vi "test_erp42.vi"(11 "Data":T3={"Drive_value"={"F/B"=enum."N", "Speed"=0, "Steer"=-82, "A/M"=enum."Auto", "Brake"=0}} {"Drive_value"."Brake" scale=0.0..200.0; "Drive_value"."Steer" scale=-2000.0..2000.0; "Drive_value"."Speed" scale=0.0..100.0}) -> (2 "ERP_Receive":T2, 3 "data val":bool)   [LabVIEW 2019]
uses:
  Ctrl/data.ctl
  Ctrl/erp42_receive_packet.ctl
panel:
  in  "AGV cfg":T1={"Port"="COM32", "speed limits"={"limit_linear-v"=0.5, "limit_angular-v"=0.7999999999999999}}
  in  "정지":bool
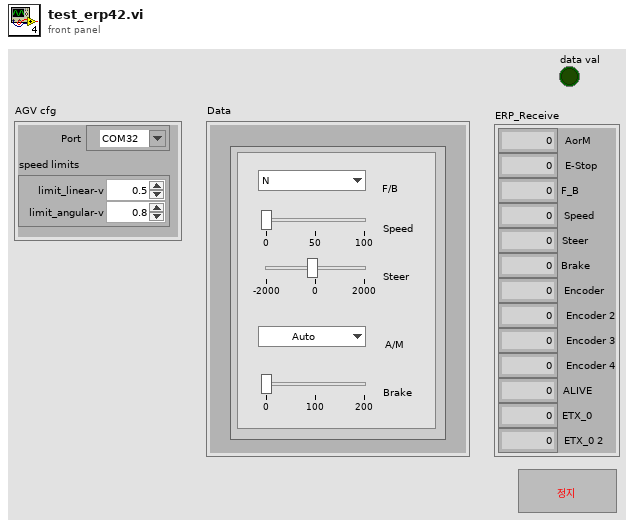
[diagram p1: front panel]
types:
  T1 = cluster{"Port":refnum<visa-resource-name>, "speed limits":cluster{"limit_linear-v":dbl, "limit_angular-v":dbl}}
  T2 = typedef "erp42_receive_packet.ctl" = cluster{"AorM":u8, "E-Stop":u8, "F_B":u8, "Speed":u16, "Steer":i16, "Brake":u8, "Encoder":u8, "Encoder 2":u8, "Encoder 3":u8, "Encoder 4":u8, "ALIVE":u8, "ETX_0":u8, "ETX_0 2":u8}
  T3 = typedef "data.ctl" = cluster{"Drive_value":cluster{"F/B":enum16{"Go", "N", "Back"}, "Speed":u16, "Steer":i16, "A/M":enum16{"Brake", "Auto", "Manual"}, "Brake":u8}}
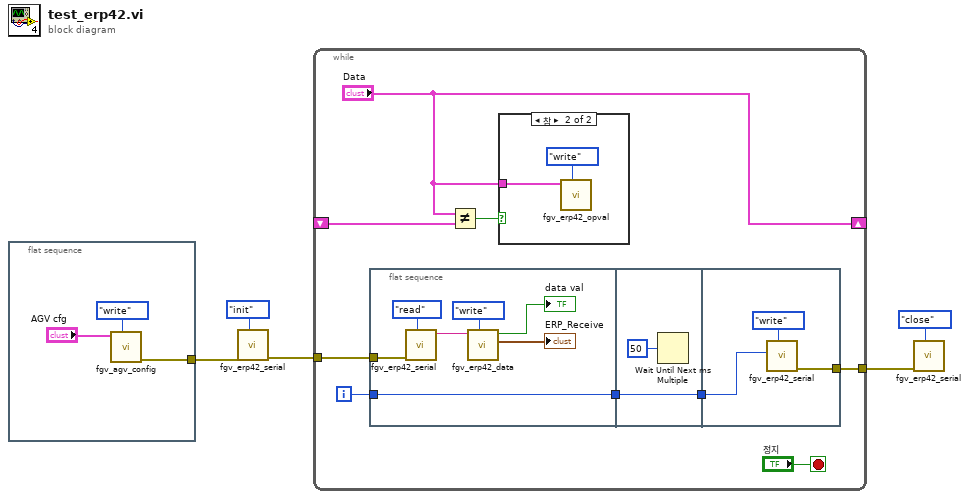
[diagram p0: block diagram]
diagram:
  n1 = flat-sequence {
    tunnel: [w8] -> w1
    frame #0 {
      n2 = call "fgv_agv_config.vi"("cmd"=enum16{"read", "write"}."write", "AGV cfg"="AGV cfg") -> ("error out"=w8:errorcluster)  [unwired: 8 in, 1 out]
    }
  }
  n3 = call "fgv_erp42_serial.vi"("cmd"=enum16{"init", "read", "write", "close"}."init", "error in"=w1) -> ("error out"=w2:errorcluster)  [unwired: 6 in, 3 out]
  n4 = while {
    tunnel: [w16] -> w3
    tunnel: w2 -> [w15]
    shift-right: ["Data"] -> _
    shift-left: _ -> [w11]
    i -> [w14]
    stop <- "정지" stop-if-true
    n5 = flat-sequence {
      tunnel: w15 -> [w25]
      tunnel: w14 -> [w24]
      tunnel: [w24] -> w13
      tunnel: w13 -> [w27]
      tunnel: [w27] -> w12
      tunnel: [w30] -> w16
      tunnel: w12 -> [w29]
      frame #0 {
        n6 = call "fgv_erp42_serial.vi"("cmd"=enum16{"init", "read", "write", "close"}."read", "error in"=w25) -> ("read_buffer"=w20:string)  [unwired: 6 in, 3 out]
        n7 = call "fgv_erp42_data.vi"("cmd"=enum16{"init", "read", "write"}."write", "erp recv str"=w20) -> ("ERP_Receive out"=→"ERP_Receive":T2, "val"=→"data val":bool)  [unwired: 7 in, 1 out]
      }
      frame #1 {
        n8 = Wait Until Next ms Multiple(millisecond multiple=u32 50 ("ms 배수")) -> ()  [unwired: 1 out]
      }
      frame #2 {
        n9 = call "fgv_erp42_serial.vi"("cmd"=enum16{"init", "read", "write", "close"}."write", "count"=w29) -> ("error out"=w30:errorcluster)  [unwired: 6 in, 3 out]
      }
    }
    n10 = Not Equal?(x="Data", y=w11) -> (x != y?=w10:bool)
    n11 = case shown="참" w10 {
      tunnel: "Data" -> [_ w18]
      frame False {
      }
      frame True {
        n12 = call "fgv_erp42_opval.vi"("cmd"=enum16{"read", "write", "ini"}."write", "data_in"=w18) -> ()  [unwired: 9 in, 1 out]
      }
    }
  }
  n13 = call "fgv_erp42_serial.vi"("cmd"=enum16{"init", "read", "write", "close"}."close", "error in"=w3) -> ()  [unwired: 6 in, 4 out]
